vi "Control - Load Command - High-Idle Governor.vi"(0 "Control Inputs":T1={"Engine Speed [RPM]"=0.0, "Engine Status"=enum."STALLED", "Load Control \nMode"=enum."High-Idle Governor", "dt(s)"=0.0, "Number of Cylinders"=0, "Engine Displacement [cc]"=0.0, "StoichAFR"=0.0, "Q.LHV Fuel [kJ/kg]"=0.0, "BattV PSU [V]"=0.0, "12V PSU [V]"=0.0, "5V PSU [V]"=0.0, "Pedal Position [%]"=0.0, "Oil Pressure [kPa]"=0.0, "Oil Temp [C]"=0.0, "Oil Level [%]"=0.0, "Engine Coolant Temp (ECT) [C]"=0.0, "Engine Coolant Pressure [kPa]"=0.0, "Rail Pressure [bar]"=0.0, "Fuel Pressure [kPa]"=0.0, "Fuel Temp [C]"=0.0, "Vacuum Pressure [kPa]"=0.0, "Throttle Position [%]"=0.0, "Cam1 Advance [CAD]"=0.0, "Cam2 Advance [CAD]"=0.0, "Cam3 Advance [CAD]"=0.0, "Cam4 Advance [CAD]"=0.0, "CA50 Control Output [CAD]"=[], "CA50 Control Output Valid"=[], "Intake Air Temp (IAT) [C]"=0.0, "Barometric Air Pressure [kPa]"=0.0, "Intake Air Rel. Humidity [%]"=0.0, "Mass Air Flow (MAF) [kg/hr]"=0.0, "Turbo Inlet Air Pressure [kPa]"=0.0, "Turbo Inlet Air Temp [C]"=0.0, "Turbo Outlet Air Pressure [kPa]"=0.0, "Turbo Outlet Air Temp [C]"=0.0, "CAC Outlet Pressure [kPa]"=0.0, "CAC Outlet Temp [C]"=0.0, "Intake Manifold Pressure (MAP) [kPa]"=0.0, "Intake Manifold Temp (MAT) [C]"=0.0, "Exhaust Manifold Pressure [kPa]"=0.0, "Exhaust Manifold Temp [C]"=0.0, "HighP EGR Cooler Outlet Pressure [kPa]"=0.0, "HighP EGR Cooler Outlet Temp [C]"=0.0, "HighP EGR Differential Pressure [kPa]"=0.0, "HighP EGR Valve Position [%]"=0.0, "Turbo Outlet Exhaust Pressure [kPa]"=0.0, "Turbo Outlet Exhaust Temp [C]"=0.0, "VGT Position 1 [%]"=0.0, "VGT Position 2 [%]"=0.0, "Turbo Speed 1 [RPM]"=0.0, "Turbo Speed 2 [RPM]"=0.0, "LowP EGR Differential Pressure [kPa]"=0.0, "LowP EGR Valve Position [%]"=0.0, "UEGO1Lambda"=0.0, "UEGO1_Hot"=FALSE, "UEGO2Lambda"=0.0, "UEGO2_Hot"=FALSE, "Knock Intensity"=[], "Knock"=[]} {"Knock Intensity" format="%.2f"; "CA50 Control Output [CAD]" format="%.2f"; "Exhaust Manifold Temp [C]" format="%#_6f"; "UEGO2Lambda" format="%.2f"; "Intake Manifold Temp (MAT) [C]" format="%#_6f"; "UEGO1Lambda" format="%.2f"}, 3 "BeatbackDiff":sgl, 4 "Pedal In":sgl, 5 "Load Control Mode In":T3) -> (7 "Governor Output":sgl, 9 "PEffort":sgl, 11 "IEffort":sgl, 13 "DEffort":sgl, 14 "Control Inputs":T1={"Engine Speed [RPM]"=0.0, "Engine Status"=enum."STALLED", "Load Control \nMode"=enum."High-Idle Governor", "dt(s)"=0.0, "Number of Cylinders"=0, "Engine Displacement [cc]"=0.0, "StoichAFR"=0.0, "Q.LHV Fuel [kJ/kg]"=0.0, "BattV PSU [V]"=0.0, "12V PSU [V]"=0.0, "5V PSU [V]"=0.0, "Pedal Position [%]"=0.0, "Oil Pressure [kPa]"=0.0, "Oil Temp [C]"=0.0, "Oil Level [%]"=0.0, "Engine Coolant Temp (ECT) [C]"=0.0, "Engine Coolant Pressure [kPa]"=0.0, "Rail Pressure [bar]"=0.0, "Fuel Pressure [kPa]"=0.0, "Fuel Temp [C]"=0.0, "Vacuum Pressure [kPa]"=0.0, "Throttle Position [%]"=0.0, "Cam1 Advance [CAD]"=0.0, "Cam2 Advance [CAD]"=0.0, "Cam3 Advance [CAD]"=0.0, "Cam4 Advance [CAD]"=0.0, "CA50 Control Output [CAD]"=[], "CA50 Control Output Valid"=[], "Intake Air Temp (IAT) [C]"=0.0, "Barometric Air Pressure [kPa]"=0.0, "Intake Air Rel. Humidity [%]"=0.0, "Mass Air Flow (MAF) [kg/hr]"=0.0, "Turbo Inlet Air Pressure [kPa]"=0.0, "Turbo Inlet Air Temp [C]"=0.0, "Turbo Outlet Air Pressure [kPa]"=0.0, "Turbo Outlet Air Temp [C]"=0.0, "CAC Outlet Pressure [kPa]"=0.0, "CAC Outlet Temp [C]"=0.0, "Intake Manifold Pressure (MAP) [kPa]"=0.0, "Intake Manifold Temp (MAT) [C]"=0.0, "Exhaust Manifold Pressure [kPa]"=0.0, "Exhaust Manifold Temp [C]"=0.0, "HighP EGR Cooler Outlet Pressure [kPa]"=0.0, "HighP EGR Cooler Outlet Temp [C]"=0.0, "HighP EGR Differential Pressure [kPa]"=0.0, "HighP EGR Valve Position [%]"=0.0, "Turbo Outlet Exhaust Pressure [kPa]"=0.0, "Turbo Outlet Exhaust Temp [C]"=0.0, "VGT Position 1 [%]"=0.0, "VGT Position 2 [%]"=0.0, "Turbo Speed 1 [RPM]"=0.0, "Turbo Speed 2 [RPM]"=0.0, "LowP EGR Differential Pressure [kPa]"=0.0, "LowP EGR Valve Position [%]"=0.0, "UEGO1Lambda"=0.0, "UEGO1_Hot"=FALSE, "UEGO2Lambda"=0.0, "UEGO2_Hot"=FALSE, "Knock Intensity"=[], "Knock"=[]} {"Knock Intensity" format="%.2f"; "CA50 Control Output [CAD]" format="%.2f"; "Exhaust Manifold Temp [C]" format="%#_6f"; "UEGO2Lambda" format="%.2f"; "Intake Manifold Temp (MAT) [C]" format="%#_6f"; "UEGO1Lambda" format="%.2f"}, 18 "Pedal Out":sgl, 19 "Load Control Mode Out":T3)   [LabVIEW 2015, in "ECS-RT.lvlib"]
doc: "This VI is a High-Idle Governor. It utilizes a Beatback PID to ensure bumpless transition. The BeatbackDiff must be supplied as an input via feedback node to utilize this feature."
uses:
  ECS-RT.lvlib
  Typedefs/Control Inputs/Control Inputs.ctl
  Typedefs/EPT/Engine Status.ctl
  Typedefs/MISC/Load Control Mode.ctl
  ECS-Shared.lvlib
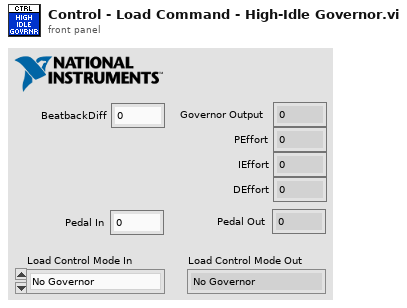
[diagram p1: front panel]
types:
  T1 = typedef "ECS-Shared.lvlib/Control Inputs.ctl" = cluster{"Engine Speed [RPM]":sgl, "Engine Status":T2, "Load Control \nMode":T3, "dt(s)":sgl, "Number of Cylinders":u8, "Engine Displacement [cc]":sgl, "StoichAFR":sgl, "Q.LHV Fuel [kJ/kg]":sgl, "BattV PSU [V]":sgl, "12V PSU [V]":sgl, "5V PSU [V]":sgl, "Pedal Position [%]":sgl, "Oil Pressure [kPa]":sgl, "Oil Temp [C]":sgl, "Oil Level [%]":sgl, "Engine Coolant Temp (ECT) [C]":sgl, "Engine Coolant Pressure [kPa]":sgl, "Rail Pressure [bar]":sgl, "Fuel Pressure [kPa]":sgl, "Fuel Temp [C]":sgl, "Vacuum Pressure [kPa]":sgl, "Throttle Position [%]":sgl, "Cam1 Advance [CAD]":sgl, "Cam2 Advance [CAD]":sgl, "Cam3 Advance [CAD]":sgl, "Cam4 Advance [CAD]":sgl, "CA50 Control Output [CAD]":sgl[], "CA50 Control Output Valid":bool[], "Intake Air Temp (IAT) [C]":sgl, "Barometric Air Pressure [kPa]":sgl, "Intake Air Rel. Humidity [%]":sgl, "Mass Air Flow (MAF) [kg/hr]":sgl, "Turbo Inlet Air Pressure [kPa]":sgl, "Turbo Inlet Air Temp [C]":sgl, "Turbo Outlet Air Pressure [kPa]":sgl, "Turbo Outlet Air Temp [C]":sgl, "CAC Outlet Pressure [kPa]":sgl, "CAC Outlet Temp [C]":sgl, "Intake Manifold Pressure (MAP) [kPa]":sgl, "Intake Manifold Temp (MAT) [C]":sgl, "Exhaust Manifold Pressure [kPa]":sgl, "Exhaust Manifold Temp [C]":sgl, "HighP EGR Cooler Outlet Pressure [kPa]":sgl, "HighP EGR Cooler Outlet Temp [C]":sgl, "HighP EGR Differential Pressure [kPa]":sgl, "HighP EGR Valve Position [%]":sgl, "Turbo Outlet Exhaust Pressure [kPa]":sgl, "Turbo Outlet Exhaust Temp [C]":sgl, "VGT Position 1 [%]":sgl, "VGT Position 2 [%]":sgl, "Turbo Speed 1 [RPM]":sgl, "Turbo Speed 2 [RPM]":sgl, "LowP EGR Differential Pressure [kPa]":sgl, "LowP EGR Valve Position [%]":sgl, "UEGO1Lambda":sgl, "UEGO1_Hot":bool, "UEGO2Lambda":sgl, "UEGO2_Hot":bool, "Knock Intensity":sgl[], "Knock":bool[]}
  T2 = typedef "ECS-Shared.lvlib/Engine Status.ctl" = enum16{"OFF", "STALLED", "CRANKING", "RUNNING", "ACCEL", "DECEL", "SAFE"}
  T3 = typedef "ECS-Shared.lvlib/Load Control Mode.ctl" = enum16{"No Governor", "Low-Idle Governor", "High-Idle Governor"}
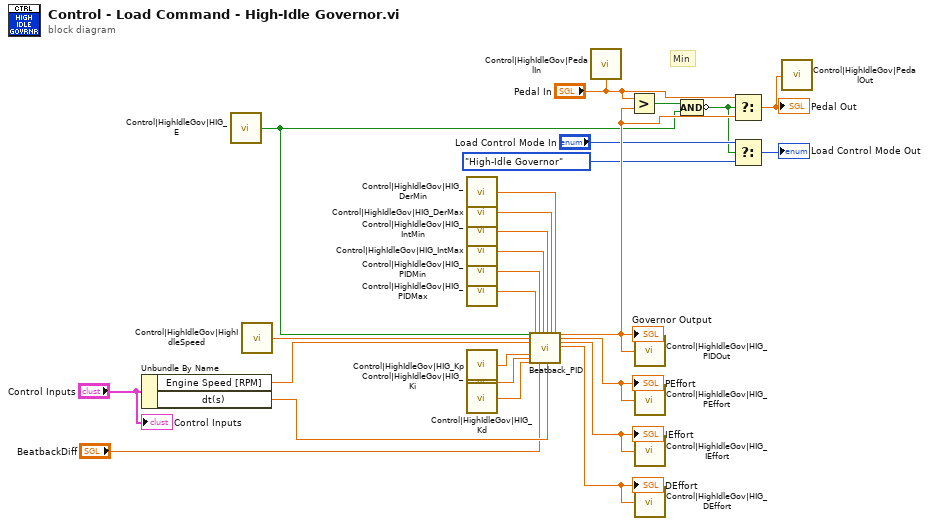
[diagram p0: block diagram]
diagram:
  # "Min"
  n1 = Unbundle By Name("Control Inputs") -> ("Engine Speed [RPM]"=w26:sgl, "dt(s)"=w17:sgl)
  n2 = call "Control|HighIdleGov|HIG_E"() -> ("Value"=w2:bool)
  n3 = call "Control|HighIdleGov|HighIdleSpeed"() -> ("Value"=w11:sgl)
  n4 = call "Control|HighIdleGov|HIG_DerMin"() -> ("Value"=w12:sgl)
  n5 = call "Control|HighIdleGov|HIG_DerMax"() -> ("Value"=w13:sgl)
  n6 = call "Control|HighIdleGov|HIG_IntMin"() -> ("Value"=w14:sgl)
  n7 = call "Control|HighIdleGov|HIG_IntMax"() -> ("Value"=w15:sgl)
  n8 = call "Control|HighIdleGov|HIG_PIDMin"() -> ("Value"=w25:sgl)
  n9 = call "Control|HighIdleGov|HIG_PIDMax"() -> ("Value"=w24:sgl)
  n10 = call "Control|HighIdleGov|HIG_Kp"() -> ("Value"=w23:sgl)
  n11 = call "Control|HighIdleGov|HIG_Ki"() -> ("Value"=w22:sgl)
  n12 = call "Control|HighIdleGov|HIG_Kd"() -> ("Value"=w21:sgl)
  n13 = call "Beatback_PID.vi"("Enable"=w2, "Setpoint"=w11, "ProcessVariable"=w26, "Kp"=w23, "Ki"=w22, "Kd"=w21, "OutLLim"=w24, "OutULim"=w25, "BeatbackDiff"="BeatbackDiff", "IntLLim"=w15, "IntULim"=w14, "dt [s]"=w17, "DerLLim"=w13, "DerULim"=w12) -> ("Output"=w10:sgl, "PEffort"=w18:sgl, "IEffort"=w20:sgl, "DEffort"=w19:sgl)  [unwired: 8 in, 2 out]
  "Governor Output" <- w10
  "PEffort" <- w18
  "IEffort" <- w20
  "DEffort" <- w19
  n14 = call "Control|HighIdleGov|PedalIn"("Value"="Pedal In") -> ()
  n15 = Greater?(x="Pedal In", y=w10) -> (0:w1:bool)
  n16 = call "Control|HighIdleGov|HIG_PIDOut"("Value"=w10) -> ()
  n17 = call "Control|HighIdleGov|HIG_PEffort"("Value"=w18) -> ()
  n18 = call "Control|HighIdleGov|HIG_IEffort"("Value"=w20) -> ()
  n19 = call "Control|HighIdleGov|HIG_DEffort"("Value"=w19) -> ()
  n20 = Compound Arithmetic op=AND(w1, w2) -> (invert w3:bool)
  n21 = Select(t="Pedal In", s=w3, f=w10) -> (s? t:f=w4:sgl)
  "Pedal Out" <- w4
  n22 = Select(t="Load Control Mode In", s=w3, f=Load_Control_Mode."High-Idle Governor" ("Load Control Mode")) -> (s? t:f=→"Load Control Mode Out":T3)
  n23 = call "Control|HighIdleGov|PedalOut"("Value"=w4) -> ()
  "Control Inputs" <- "Control Inputs"
